vi "并道从数组读取.vi"(1 "并道":enum16{"8192道", "4096道", "2048道", "1024道"}(ring), 2 "数组":i32[](array[numeric])) -> (0 "波形图":i32[](graph))   [LabVIEW 2014]
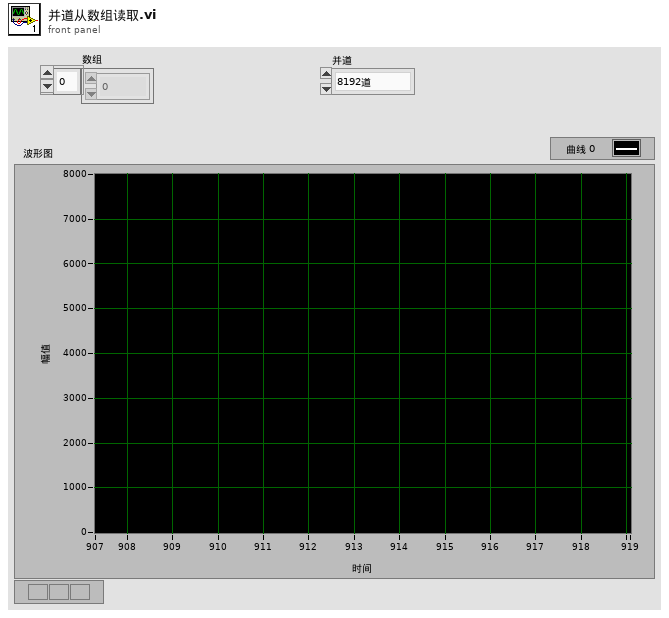
[diagram p1: front panel]
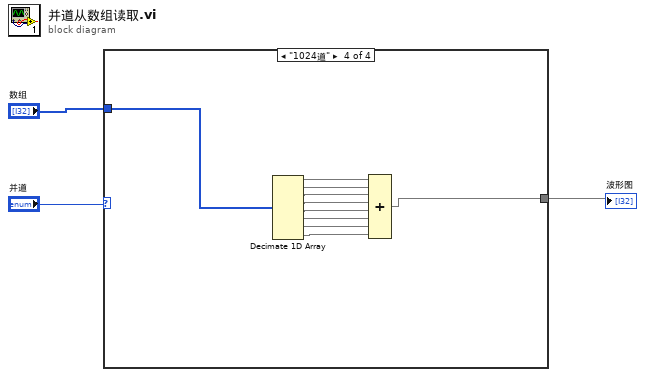
[diagram p0: block diagram]
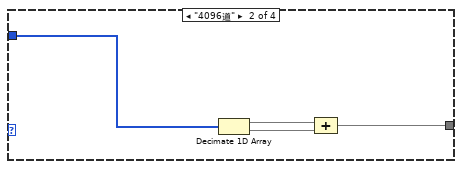
[diagram p3: hidden frame]
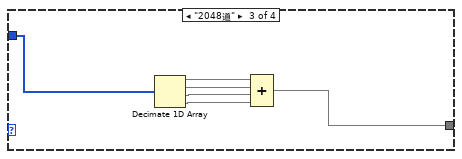
[diagram p4: hidden frame]
diagram:
  n1 = case shown="\"1024道\"" "并道" {
    tunnel: "数组" -> [w4 w8 w10 w16]
    tunnel: [w4 w5 w9 w15] -> w2
    frame "8192道", Default {
    }
    frame "4096道" {
      n2 = Decimate 1D Array(w8) -> (w7:i32[], w6:i32[])
      n3 = Compound Arithmetic op=ADD(w7, w6) -> (w5:i32[])
    }
    frame "2048道" {
      n4 = Decimate 1D Array(w10) -> (w14:i32[], w13:i32[], w12:i32[], w11:i32[])
      n5 = Compound Arithmetic op=ADD(w14, w13, w12, w11) -> (w9:i32[])
    }
    frame "1024道" {
      n6 = Decimate 1D Array(w16) -> (w24:i32[], w23:i32[], w22:i32[], w21:i32[], w20:i32[], w19:i32[], w18:i32[], w17:i32[])
      n7 = Compound Arithmetic op=ADD(w24, w23, w22, w21, w20, w19, w18, w17) -> (w15:i32[])
    }
  }
  "波形图" <- w2
